vi "PXI-4130 Configure DCpwr (RT).vi"(8 "error in (no error)":errorcluster, 11 "Item Ref in":T1 format="%.0x") -> (0 "error out":errorcluster, 1 "Channel 1 Type":i32, 2 "Channel 0 Type":i32, 3 "Item Ref out":T1 format="%.0x", 5 "instrument handle out":refnum<k15>)   [LabVIEW 2009, in "PXI-4130 Custom Device.lvlib"]
uses:
  PXI-4130 Custom Device.lvlib
  <vilib>/NI VeriStand/Custom Device API/Custom Device Item Ref.ctl
  <vilib>/NI VeriStand/Custom Device API/Get Item Property (I32).vi
  <vilib>/NI VeriStand/Custom Device API/Get Item Property (String).vi
  PXI-4130 Global Variable.vi
  <instrlib>/niDCPower/nidcpower.llb/niDCPower Source Mode.ctl
  <vilib>/NI VeriStand/Custom Device API/Custom Device API.lvlib
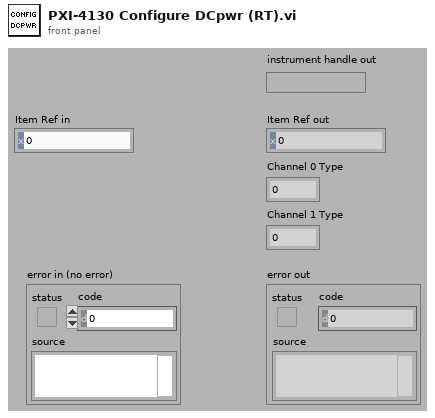
[diagram p1: front panel]
types:
  T1 = typedef "Custom Device API.lvlib/Custom Device Item Ref.ctl" = u64
  T2 = typedef "niDCPower Source Mode.ctl" = i32
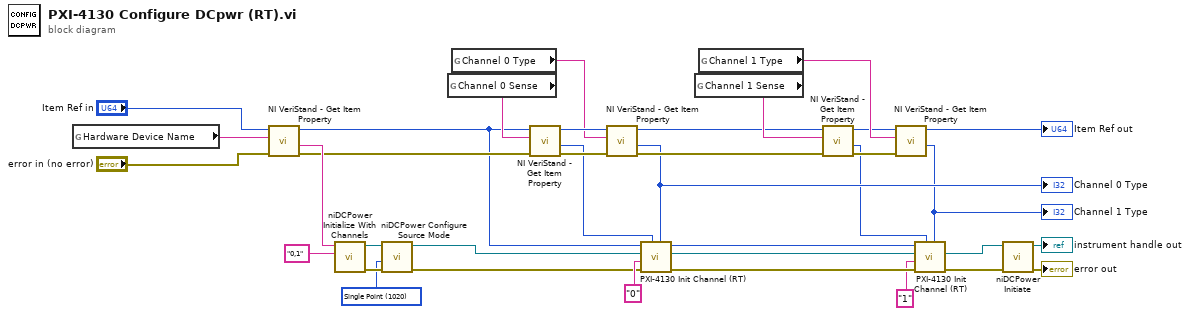
[diagram p0: block diagram]
diagram:
  w9 = T2 1020 items=["Single Point"=1020, "Sequence"=1021] ("source mode")
  n1 = global read "PXI-4130 Global Variable.vi" "Hardware Device Name"() -> (w36:string)
  n2 = call-poly <vilib>:"NI VeriStand - Get Item Property.vi"("error in (no error)"="error in (no error)", "Property Name"=w36, "Item Ref in"="Item Ref in") -> ("error out"=w32:errorcluster, "Value"=w35:string, "Item Ref out"=w17:T1)  [unwired: 5 in, 1 out]
  n3 = call <instrlib>:"niDCPower Initialize With Channels.vi"("channels"="0,1", "resource name"=w35) -> ("error out"=w11:errorcluster, "instrument handle out"=w13:refnum<k15>)  [unwired: 8 in]
  n4 = call <instrlib>:"niDCPower Configure Source Mode.vi"("error in (no error)"=w11, "source mode"=w9, "instrument handle"=w13) -> ("error out"=w10:errorcluster, "instrument handle out"=w12:refnum<k15>)  [unwired: 7 in]
  n5 = global read "PXI-4130 Global Variable.vi" "Channel 0 Sense"() -> (w30:string)
  n6 = global read "PXI-4130 Global Variable.vi" "Channel 0 Type"() -> (w29:string)
  n7 = call-poly <vilib>:"NI VeriStand - Get Item Property.vi"("error in (no error)"=w32, "Property Name"=w30, "Item Ref in"=w17) -> ("error out"=w31:errorcluster, "Value"=w22:i32, "Item Ref out"=w33:T1)  [unwired: 5 in, 1 out]
  n8 = call-poly <vilib>:"NI VeriStand - Get Item Property.vi"("error in (no error)"=w31, "Property Name"=w29, "Item Ref in"=w33) -> ("error out"=w23:errorcluster, "Value"=w21:i32, "Item Ref out"=w24:T1)  [unwired: 5 in, 1 out]
  "Channel 0 Type" <- w21
  n9 = call "PXI-4130 Init Channel (RT).vi"("Channel Type"=w21, "Channel Sense"=w22, "error in (no error)"=w10, "Channel Name"="0", "resource name"=w12, "Device Reference In"=w17) -> ("error out"=w18:errorcluster, "resource name Out"=w14:refnum<k15>, "Device Reference Out"=w20:T1)  [unwired: 3 in]
  n10 = global read "PXI-4130 Global Variable.vi" "Channel 1 Sense"() -> (w28:string)
  n11 = global read "PXI-4130 Global Variable.vi" "Channel 1 Type"() -> (w27:string)
  n12 = call-poly <vilib>:"NI VeriStand - Get Item Property.vi"("error in (no error)"=w23, "Property Name"=w28, "Item Ref in"=w24) -> ("error out"=w25:errorcluster, "Value"=w19:i32, "Item Ref out"=w26:T1)  [unwired: 5 in, 1 out]
  n13 = call-poly <vilib>:"NI VeriStand - Get Item Property.vi"("error in (no error)"=w25, "Property Name"=w27, "Item Ref in"=w26) -> ("Value"=w8:i32, "Item Ref out"=→"Item Ref out":T1)  [unwired: 5 in, 2 out]
  "Channel 1 Type" <- w8
  n14 = call "PXI-4130 Init Channel (RT).vi"("Channel Type"=w8, "Channel Sense"=w19, "error in (no error)"=w18, "Channel Name"="1", "resource name"=w14, "Device Reference In"=w20) -> ("error out"=w6:errorcluster, "resource name Out"=w7:refnum<k15>)  [unwired: 3 in, 1 out]
  n15 = call <instrlib>:"niDCPower Initiate.vi"("error in (no error)"=w6, "instrument handle"=w7) -> ("error out"=→"error out":errorcluster, "instrument handle out"=→"instrument handle out":refnum<k15>)  [unwired: 8 in]
